vi "Keep Max.vi"(7 "Reset(F)":bool, 11 "Value":dbl) -> (3 "Average":dbl)   [LabVIEW 2017]
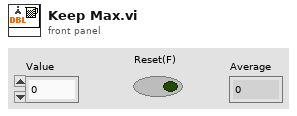
[diagram p1: front panel]
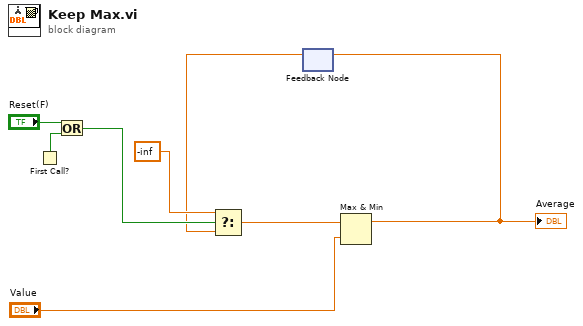
[diagram p0: block diagram]
diagram:
  n1 = First Call?() -> (First Call?: T/F=w7:bool)
  n2 = Or(x="Reset(F)", y=w7) -> (x .or. y?=w6:bool)
  n3 = feedback #1() -> (w1:dbl)  [unwired: 1 in]
  n4 = Select(t=-inf, s=w6, f=w1) -> (s? t:f=w4:dbl)
  n5 = Max & Min(x=w4, y="Value") -> (max(x,y)=w2:dbl)  [unwired: 1 out]
  "Average" <- w2
  n6 = feedback-in #1(w2) -> ()
